vi "main.vi"() -> ()   [LabVIEW 2023]
uses:
  pico_scpi_labtool_labview_driver/scpi_driver/usbtmc_scpi_labtool.lvlib
panel:
  in  "Python Loop":bool
  out "return value":string
  in  "function name":string
  in  "module path":path
  in  "Python error in":errorcluster
  in  "Python version":string
  in  "Relay Control Pin":u8 max=7 step=1
  out "Duty Cycle":dbl
  out "Temp threshold crossed":bool
  in  "Temperature Read":u8 max=7 step=1
  in  "Duty Cycle Control":u8 max=7 step=1
  out "RPM":dbl(knob) scale=0.0..10000.0
  in  "RPM Loop":bool
  out "Waveform Chart":i32(graph)
  in  "RPM sensor data Pin":u8 max=7 step=1
  in  "VISA error in":errorcluster caption="error in (no error)"
  in  "VISA resource name in":refnum<visa-resource-name>
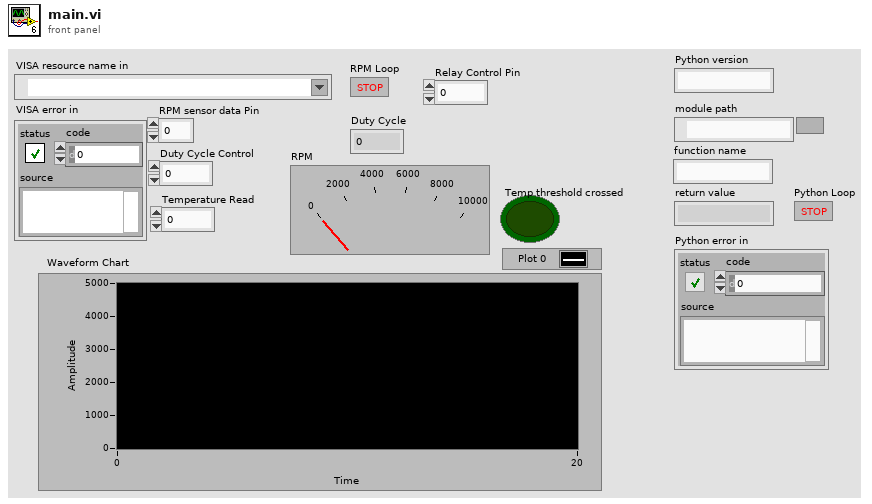
[diagram p1: front panel]
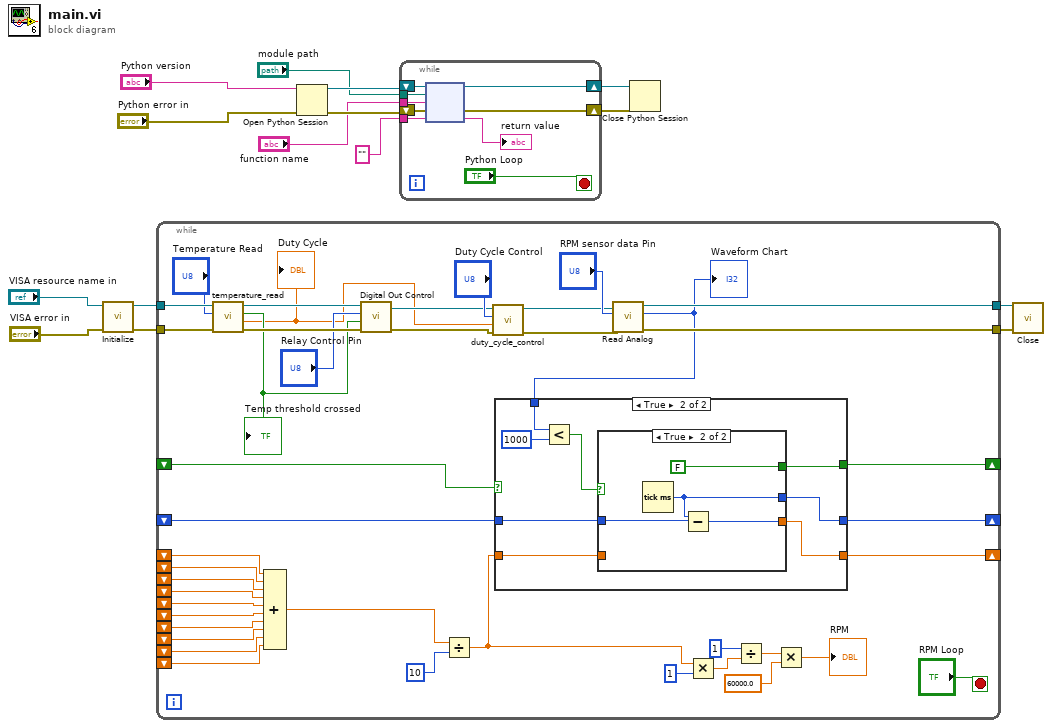
[diagram p0: block diagram]
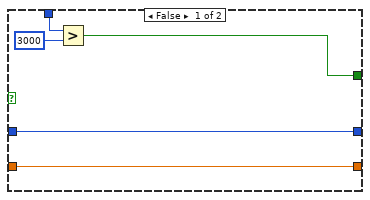
[diagram p2: hidden frame]
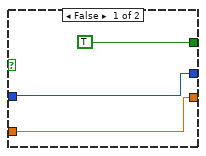
[diagram p3: hidden frame]
diagram:
  n1 = call "Initialize.vi"("error in (no error)"="VISA error in", "VISA resource name in"="VISA resource name in") -> ("error out"=w11:errorcluster, "VISA resource name out"=w10:refnum<visa-resource-name>)  [unwired: 8 in]
  n2 = while {
    tunnel: [w57] -> w13
    tunnel: [w56] -> w12
    shift-right: [w53] -> _
    shift-left: _ -> [w52]
    shift-right: [w51] -> _
    shift-left: _ -> [w50]
    shift-right: [w43] -> _
    shift-left: _ -> [w42]
    shift-left: _ -> [w41]
    shift-left: _ -> [w40]
    shift-left: _ -> [w39]
    shift-left: _ -> [w38]
    shift-left: _ -> [w33]
    shift-left: _ -> [w34]
    shift-left: _ -> [w35]
    shift-left: _ -> [w36]
    shift-left: _ -> [w37]
    tunnel: w11 -> [w25]
    tunnel: w10 -> [w26]
    stop <- "RPM Loop" stop-if-true
    n3 = call "temperature_read.vi"("error in (no error)"=w25, "Pin"="Temperature Read", "VISA resource name"=w26) -> ("error out"=w20:errorcluster, "Duty Cycle (%)"=w16:dbl, "Temp threshold crossed"=w17:bool, "VISA resource name out"=w22:refnum<visa-resource-name>)  [unwired: 5 in]
    "Temp threshold crossed" <- w17
    "Duty Cycle" <- w16
    n4 = Compound Arithmetic op=ADD(w42, w41, w40, w39, w38, w33, w34, w35, w36, w37) -> (w32:dbl)
    n5 = call "Digital Out Control.vi"("VISA resource name"=w22, "Pin"="Relay Control Pin", "Enable Pin (F: Off)"=w17, "error in (no error)"=w20) -> ("VISA resource name out"=w21:refnum<visa-resource-name>, "error out"=w19:errorcluster)  [unwired: 5 in]
    n6 = Divide(x=w32, y=u32 10) -> (x/y=w30:dbl)
    n7 = call "duty_cycle_control.vi"("error in (no error)"=w19, "Duty Cycle (%)"=w16, "Pin"="Duty Cycle Control", "VISA resource name"=w21) -> ("error out"=w29:errorcluster, "VISA resource name out"=w28:refnum<visa-resource-name>)  [unwired: 6 in]
    n8 = call "Read Analog.vi"("error in (no error)"=w29, "Pin"="RPM sensor data Pin", "VISA resource name"=w28) -> ("error out"=w56:errorcluster, "analog out"=w23:i32, "VISA resource name out"=w57:refnum<visa-resource-name>)  [unwired: 6 in]
    "Waveform Chart" <- w23
    n9 = case shown="True" w52 {
      tunnel: w23 -> [w60 w65]
      tunnel: [w58 w70] -> w53
      tunnel: [w62 w69] -> w51
      tunnel: w50 -> [w62 w68]
      tunnel: [w61 w67] -> w43
      tunnel: w30 -> [w61 w66]
      frame False {
        n10 = Greater?(x=w60, y=3000) -> (0:w58:bool)
      }
      frame True {
        n11 = Less?(x=w65, y=1000) -> (x < y?=w63:bool)
        n12 = case shown="True" w63 {
          tunnel: [TRUE FALSE] -> w70
          tunnel: [w72 w75] -> w69
          tunnel: w68 -> [w72 w76]
          tunnel: [w71 w74] -> w67
          tunnel: w66 -> [w71 _]
          frame False {
          }
          frame True {
            n13 = Tick Count (ms)() -> (millisecond timer value=w75:u32)
            n14 = Subtract(x=w75, y=w76) -> (x-y=w74:u32)
          }
        }
      }
    }
    n15 = Multiply(x=w30, y=u32 1) -> (x*y=w48:dbl)
    n16 = Divide(x=u32 1, y=w48) -> (x/y=w46:dbl)
    n17 = Multiply(x=w46, y=60000.0) -> (x*y=→"RPM":dbl)
  }
  n18 = Open Python Session(python version="Python version", 3:"Python error in") -> (session out=w7:refnum<k35>, error out=w6:errorcluster)  [unwired: 1 in]
  n19 = while {
    tunnel: "module path" -> [w82]
    tunnel: "function name" -> [w81]
    tunnel: "" -> [w80]
    shift-right: [w84] -> w5
    shift-left: w7 -> [w86]
    shift-right: [w83] -> w4
    shift-left: w6 -> [w85]
    stop <- "Python Loop" stop-if-true
    n20 = node(w86, w82, w81, w85, w80) -> (w84:refnum<k35>, w83:errorcluster, →"return value":string)  [unwired: 2 out]
  }
  n21 = Close Python Session(session in=w5, error in=w4) -> ()  [unwired: 1 out]
  n22 = call "Close.vi"("error in (no error)"=w12, "VISA resource name"=w13) -> ()  [unwired: 10 in]
